vi "LightSensorEventCreate.vi"(8 "error in (no error)":errorcluster, 11 "Devices In":u64[](array[numeric])) -> (0 "error out":errorcluster, 2 "Event Registration Refnum":refnum<event-registration>, 3 "Devices Out":u64[](array[numeric]))   [LabVIEW 2012, in "Phidget Light Sensor.lvlib"]
doc: "${IlluminanceChange:CreateHeader}"
uses:
  <instrlib>/Phidgets/Phidget Light Sensor/Phidget Light Sensor.lvlib
  <instrlib>/Phidgets/Phidget Common/Phidget Common.lvlib
  phidget22.dll
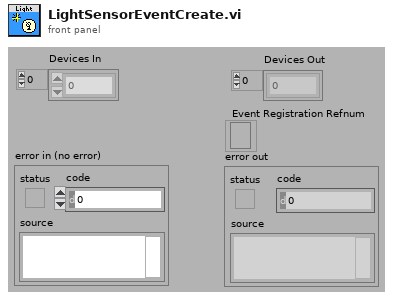
[diagram p1: front panel]
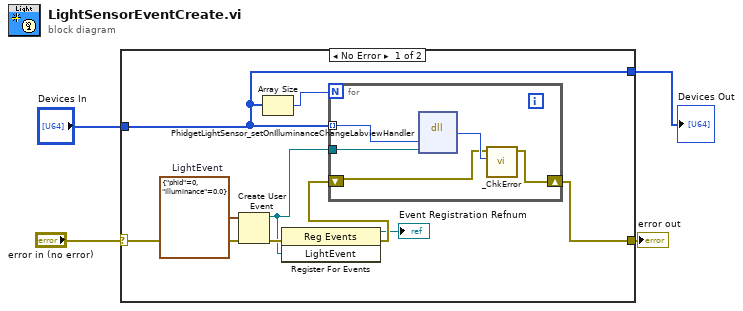
[diagram p0: block diagram]
diagram:
  n1 = case shown="No Error" "error in (no error)" {
    selector: "error in (no error)" -> [w13 w20]
    tunnel: [w9 w20] -> w3
    tunnel: "Devices In" -> [w11 w19]
    tunnel: [w11 w19] -> w1
    frame No Error {
      w7 = cluster{"phid":u64, "Illuminance":dbl} {"phid"=0, "Illuminance"=0.0}  # LightEvent
      n2 = Create User Event(user event datatype=w7, error in=w13) -> (user event=w6:refnum<user-event>, error out=w12:errorcluster)
      n3 = Array Size(array=w11) -> (size(s)=w8:i32)
      n4 = register-events(error in=w12, w6) -> (reference out=→"Event Registration Refnum":refnum<event-registration>, error out=w10:errorcluster)  [unwired: 1 in]
      n5 = for {
        N: w8 -> [_]
        tunnel: w11 -> [w16] mode=indexing
        shift-right: [w18] -> w9
        shift-left: w10 -> [w15]
        tunnel: w6 -> [w14]
        n6 = dll-call lib="phidget22.*" fn="PhidgetLightSensor_setOnIlluminanceChangeLabviewHandler"("phid"=w16, "AcceEvent"=w14) -> ("return type"=w17:i32)  [unwired: 5 in, 2 out]
        n7 = call <instrlib>:"_ChkError.vi"("Return Code"=w17, "error in (no error)"=w15) -> ("error out"=w18:errorcluster)  [unwired: 9 in]
      }
    }
    frame Error {
    }
  }
  "error out" <- w3
  "Devices Out" <- w1
